vi "All LVProj.vi"(10 "Folder":path) -> (2 "All LVProj":path[](array[path]))   [LabVIEW 2020, in "GPackTools.lvlib"]
uses:
  GPackTools.lvlib
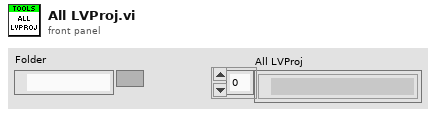
[diagram p1: front panel]
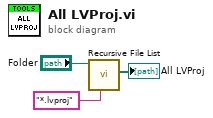
[diagram p0: block diagram]
diagram:
  n1 = call <vilib>:"Recursive File List.vi"("pattern"="*.lvproj", "Folder Path"="Folder") -> ("All Files in Dir"=→"All LVProj":path[])  [unwired: 5 in, 4 out]
